vi "TDT-Globals.vi"() -> ()   [LabVIEW 2020]
panel:
  out "in use":bool
  out "Ramp":bool
  in  "aiPos":i32
  out "TDevAccX":refnum<k7>
  out "TDT Abort":bool
  out "ZBUSx":refnum<k7>
  out "RPcox":refnum<k7>
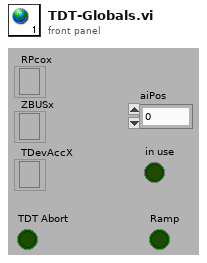
[diagram p1: front panel]
diagram:
